vi "MultiChannelFeedbackCooling_aod_feedback(Host)_PIDXYZ.vi"(5 "RIO Device":T1="RIO0") -> ()   [LabVIEW 2016]
doc: "This VI will will initialize the FPGA VI and then continually read and convert single point values from 4 channels of an analog input module."
uses:
  <vilib>/userdefined/High Color/nirio_resource_hc.ctl
  <vilib>/rvi/Analysis/host/Butterworth/config/Butterworth Filter Order.ctl
  <vilib>/rvi/Analysis/host/Butterworth/config/Butterworth Filter Type.ctl
  <vilib>/FPGAPlugInAG/PXIe-7847R/niLvFpga_Open_PXIe-7847R.vi
  <vilib>/FPGAPlugInAG/PXIe-7847R/niLvFpga_Run_PXIe-7847R.vi
  <vilib>/rvi/Analysis/host/Butterworth/config/BwScaledCoefficients.vi
  <vilib>/Utility/error.llb/Error Cluster From Error Code.vi
  <vilib>/rvi/errors/niLvFpgaAdjustHostInterfaceError.vi
  <vilib>/Utility/file.llb/Read From Spreadsheet File (I64).vi
  <vilib>/FPGAPlugInAG/PXIe-7847R/niLvFpga_Close_PXIe-7847R.vi
  <vilib>/rvi/interface/nirviOpenFPGA/nirviOpenFPGA.xnode
  FPGA Bitfiles/Microspherefeedb_FPGATarget_MultiChannelfFee_cW1Hvxk6p+4.lvbitx
  <vilib>/rvi/interface/nirviMethod/nirviMethod.xnode
  <vilib>/rvi/Analysis/host/Butterworth/XNode/ButterworthCoefficients.xnode
  <vilib>/rvi/interface/nirviReadWriteControl/nirviReadWriteControl.xnode
  <vilib>/rvi/interface/nirviCloseFPGA/nirviCloseFPGA.xnode
  NiFpgaLv.dll
  <vilib>/rvi/Analysis/host/Public/NI_FpgaMspHost.lvlib
panel:
  in  "hp freq band imgZ":dbl=5000.0
  in  "lp freq band imgZ":dbl=5000.0
  in  "dg band imgZ":fxp<+/-,24,12>
  in  "hp freq band d2Z":dbl=5000.0
  in  "lp freq band d2Z":dbl=5000.0
  in  "dg band d2Z":fxp<+/-,24,12>
  in  "hp freq bandZ":dbl=49.0
  in  "lp freq bandZ":dbl=45.0
  in  "dg band Z":fxp<+/-,24,12>
  in  "dg band Y":fxp<+/-,24,12>
  in  "hp freq bandY":dbl=5000.0
  in  "lp freq bandY":dbl=5000.0
  in  "hp freq bandX":dbl=5000.0
  in  "lp freq bandX":dbl=5000.0
  in  "dg band X":fxp<+/-,24,12>
  in  "pg 1":fxp<+/-,24,12>
  in  "ig 1":fxp<+/-,24,6>
  in  "pg 0":fxp<+/-,24,12>
  in  "ig 0":fxp<+/-,24,6>
  out "tot_fb_img":i16(graph)
  out "fb_img":i16(graph)
  out "AI_img":i16(graph)=465
  in  "pg_img":fxp<+/-,24,12>
  in  "dg_img":fxp<+/-,24,12>
  in  "ig_img":fxp<+/-,24,6>
  in  "setpt_img":i16=3000
  in  "Upper lim_img":fxp<+/-,16,16>=1000.0
  in  "Lower lim_img":fxp<+/-,16,16>=-1000.0
  in  "lp freq_img":dbl=5000.0
  in  "hp freq_img":dbl=5000.0
  in  "output offset_img":i16
  in  "End value arb (ch1)":fxp<+/-,32,16>
  in  "Step arb (ch1)":fxp<+/-,32,16>=0.0500030517578125
  in  "Arb gain (ch2)":fxp<+/-,24,12>
  in  "z arb scale":fxp<+/-,33,17>=1.0
  in  "ramp arb drive":bool
  in  "End value arb (ch0)":fxp<+/-,32,16>
  in  "Step arb (ch0)":fxp<+/-,32,16>
  in  "Delay Time (s) arb":dbl=0.001 caption="Delay Time (s)"
  in  "Buffer file path":path=path "C:/Users/UsphereLab/Documents/GitHub/Optlev/scriptssiny_buffer.txt"
  in  "Write data to buffers":bool
  in  "Arb steps per cycle":u16=50
  in  "Arb gain (ch1)":fxp<+/-,24,12>
  in  "Arb gain (ch0)":fxp<+/-,24,12>
  in  "power setpt":i16
  in  "Upper lim pow":fxp<+/-,16,16>=10000.0
  in  "Lower lim pow":fxp<+/-,16,16>=-10000.0
  in  "hp freq pow":dbl=5000.0
  in  "lp freq pow":dbl=5000.0
  in  "Use_PID2_power":bool
  in  "hp freq 1":dbl=400.0
  in  "hp freq 0":dbl=600.0
  in  "lp freq 0":dbl=600.0
  in  "DC offset 0":i16
  in  "Lower lim 0":fxp<+/-,16,16>=-200.0
  in  "Upper lim 0":fxp<+/-,16,16>=200.0
  in  "Dg 0":fxp<+/-,24,12>
  in  "Bead setpt 0":i16
  in  "change pars":bool
  in  "hp freq 2":dbl=1600.0
  in  "lp freq 1":dbl=400.0
  in  "lp freq 2":dbl=1600.0
  in  "ramp power":bool
  in  "End value power":i16=-500
  in  "Step power":i16=1
  in  "Delay Time (s) power":dbl=0.01 caption="Delay Time (s)"
  in  "Count(usec)":u32=10
  in  "?":u16(ring)=2 items=["Both", "AOD", "Bead"]
  in  "?":u16(ring)=2 items=["Both", "AOD", "Bead"]
  in  "?":u16(ring) items=["Both", "AOD", "Bead"]
  in  "?":u16(ring)=2 items=["Both", "AOD", "Bead"]
  in  "?":u16(ring)=1 items=["Both", "AOD", "Bead"]
  in  "?":u16(ring)=2 items=["Both", "AOD", "Bead"]
  in  "Pg d2":fxp<+/-,24,12>=-6.0
  in  "Ig d2":fxp<+/-,24,6>=-0.7999992370605469
  in  "Dg d2":fxp<+/-,24,12>
  in  "Ig 2":fxp<+/-,24,6>
  in  "DC offset 2":i16=2200
  in  "Lower lim 2":fxp<+/-,16,16>=-20.0
  in  "Upper lim 2":fxp<+/-,16,16>=1500.0
  in  "Dg 2":fxp<+/-,24,12>
  in  "Pg 2":fxp<+/-,24,12>
  in  "Bead setpt 2":i16
  in  "change pars 2":bool
  in  "change pars 1":bool
  in  "DC offset 1":i16
  in  "Lower lim 1":fxp<+/-,16,16>=-200.0
  in  "Upper lim 1":fxp<+/-,16,16>=200.0
  in  "Dg 1":fxp<+/-,24,12>
  in  "Bead setpt 1":i16
  out "Tot feedback + DC, Ch2":i16(graph)=2200
  out "Individual feedback, Ch2":cluster{"fb_0":i16, "fb_d0":i16}(graph)
  out "AI1 2":cluster{"AI2":i16, "AI5":i16}(graph)={"AI2"=-987, "AI5"=-987}
  out "Tot feedback + DC, Ch1":i16(graph)
  out "Individual feedback, Ch1":cluster{"fb_0":i16, "fb_d0":i16}(graph)
  out "AI1":cluster{"AI1":i16, "AI4":i16}(graph)={"AI1"=-51, "AI4"=-51}
  out "Tot feedback + DC, Ch0":i16(graph)
  out "Individual feedback, Ch0":cluster{"fb_0":i16, "fb_d0":i16}(graph)
  out "AI0":cluster{"AI0":i16, "AI3":i16}(graph)={"AI0"=-20, "AI3"=-20}
  in  "stop":bool
  # "FPGA feedback GUI"
  # "Bead arbitrary drive:"
  # "PID controls, X (ch 0):"
  # "Bead feedback:"
  # "PID controls, Y (ch 1):"
  # "Bead feedback:"
  # "PID controls, Z (ch 2):"
  # "Bead feedback:"
  # "AOD feeback:"
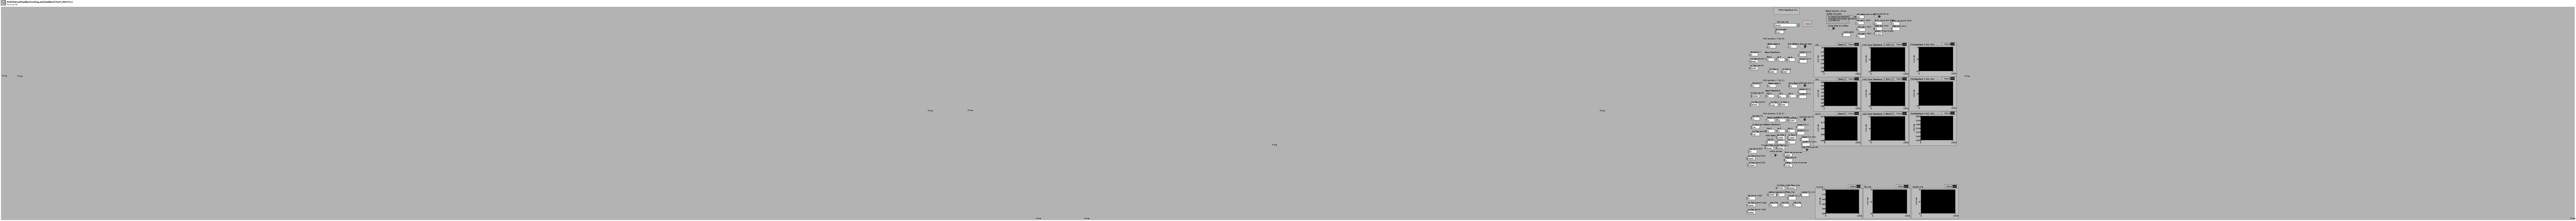
[diagram p1: front panel]
types:
  T1 = typedef "nirio_resource_hc.ctl" = tag
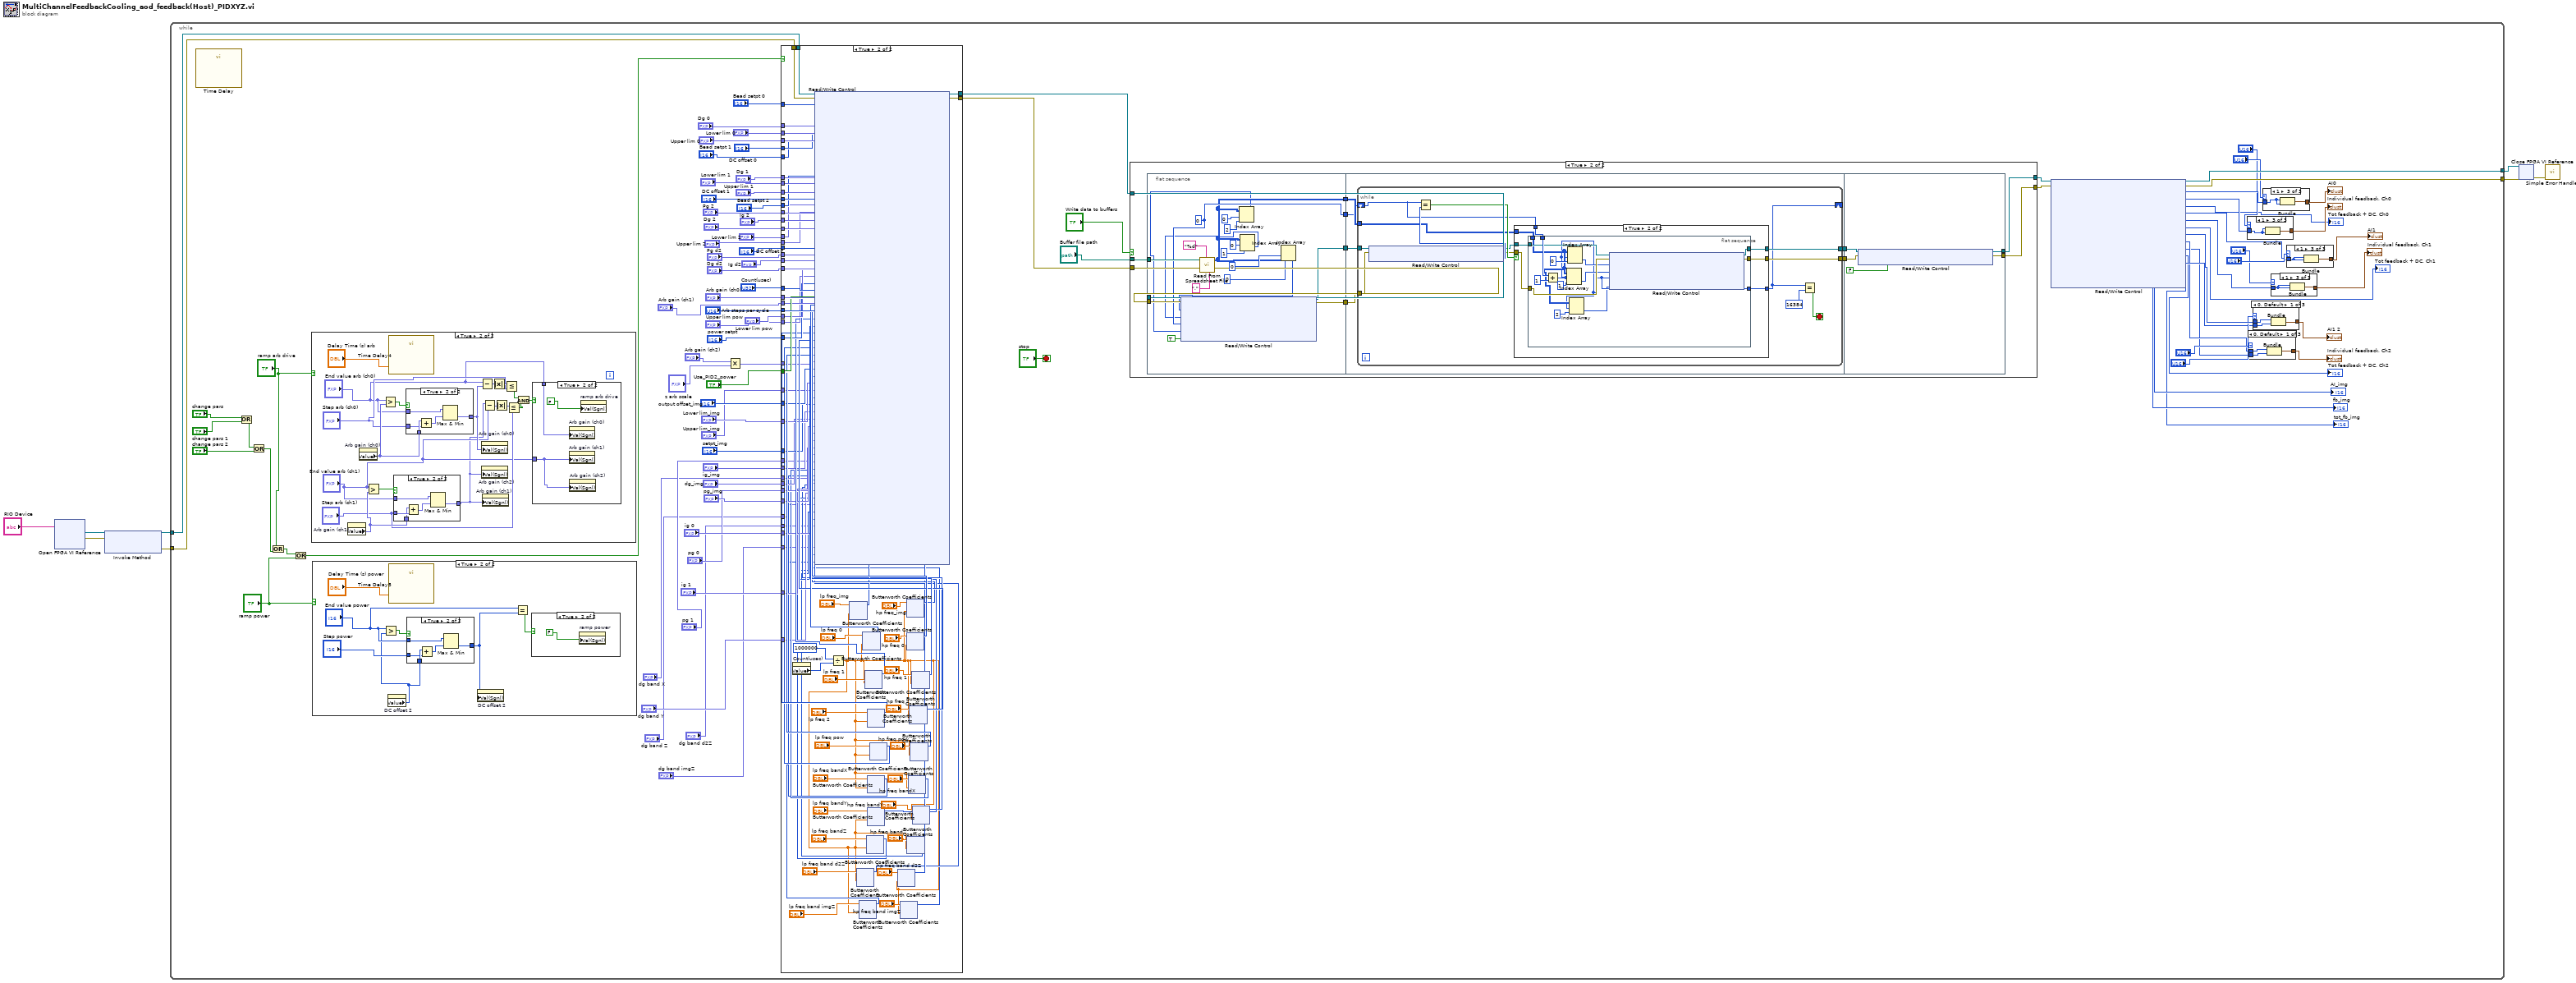
[diagram p0: block diagram]
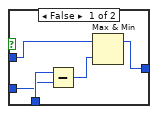
[diagram p4: hidden frame]
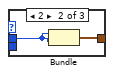
[diagram p5: hidden frame]
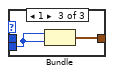
[diagram p6: hidden frame]
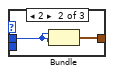
[diagram p7: hidden frame]
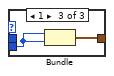
[diagram p8: hidden frame]
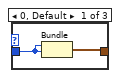
[diagram p9: hidden frame]
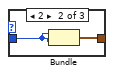
[diagram p10: hidden frame]
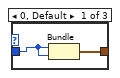
[diagram p11: hidden frame]
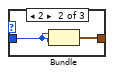
[diagram p12: hidden frame]
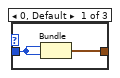
[diagram p13: hidden frame]
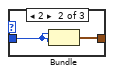
[diagram p14: hidden frame]
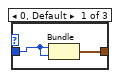
[diagram p15: hidden frame]
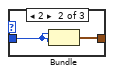
[diagram p16: hidden frame]
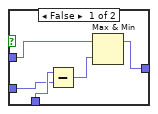
[diagram p18: hidden frame]
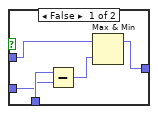
[diagram p20: hidden frame]
diagram:
  n1 = xnode "Open FPGA VI Reference"("resource name"="RIO Device") -> ("FPGA VI Reference Out"=w3:refnum<k20>, "error out"=w2:errorcluster)  [unwired: 1 in]
  n2 = xnode "Invoke Method"("FPGA VI Reference In"=w3, "error in"=w2) -> ("FPGA VI Reference Out"=w5:refnum<k20>, "error out"=w4:errorcluster)  [unwired: 1 in]
  n3 = while {
    tunnel: [w101] -> w8
    tunnel: w5 -> [w93]
    tunnel: w4 -> [w92]
    tunnel: [w100] -> w1
    stop <- "stop" stop-if-true
    n4 = call "Time Delay"() -> ()  [unwired: 11 in, 1 out]
    n5 = Or(x="change pars", y="change pars 1") -> (x .or. y?=w66:bool)
    n6 = Or(x=w66, y="change pars 2") -> (x .or. y?=w32:bool)
    n7 = Or(x="ramp arb drive", y=w32) -> (x .or. y?=w39:bool)
    n8 = Or(x=w39, y="ramp power") -> (x .or. y?=w40:bool)
    n9 = case shown="True" "ramp arb drive" {
      frame False {
      }
      frame True {
        n10 = property on="Arb gain (ch1)" class="DigNum (strict)"() -> ("Value"=w171:fxp<+/-,24,12>)  [unwired: 2 in, 2 out]
        n11 = property on="Arb gain (ch0)" class="DigNum (strict)"() -> ("Value"=w174:fxp<+/-,24,12>)  [unwired: 2 in, 2 out]
        n12 = Greater?(x="End value arb (ch1)", y=w171) -> (0:w172:bool)
        n13 = Greater?(x="End value arb (ch0)", y=w174) -> (0:w175:bool)
        n14 = call "Time Delay4"("Delay Time (s)"="Delay Time (s) arb") -> ()  [unwired: 10 in, 1 out]
        n15 = case shown="True" w172 {
          tunnel: "End value arb (ch1)" -> [w177 w183]
          tunnel: w171 -> [w180 w181]
          tunnel: "Step arb (ch1)" -> [w179 w185]
          tunnel: [w176 w182] -> w158
          frame False {
            n16 = Subtract(x=w180, y=w179) -> (x-y=w178:fxp<+/-,33,17>)
            n17 = Max & Min(x=w177, y=w178) -> (max(x,y)=w176:fxp<+/-,33,17>)  [unwired: 1 out]
          }
          frame True {
            n18 = Add(x=w181, y=w185) -> (x+y=w184:fxp<+/-,33,17>)
            n19 = Max & Min(x=w183, y=w184) -> (min(x,y)=w182:fxp<+/-,33,17>)  [unwired: 1 out]
          }
        }
        n20 = case shown="True" w175 {
          tunnel: "End value arb (ch0)" -> [w190 w195]
          tunnel: w174 -> [w193 w198]
          tunnel: "Step arb (ch0)" -> [w192 w197]
          tunnel: [w189 w194] -> w170
          frame False {
            n21 = Subtract(x=w193, y=w192) -> (x-y=w191:fxp<+/-,33,17>)
            n22 = Max & Min(x=w190, y=w191) -> (max(x,y)=w189:fxp<+/-,33,17>)  [unwired: 1 out]
          }
          frame True {
            n23 = Add(x=w198, y=w197) -> (x+y=w196:fxp<+/-,33,17>)
            n24 = Max & Min(x=w195, y=w196) -> (min(x,y)=w194:fxp<+/-,33,17>)  [unwired: 1 out]
          }
        }
        n25 = Subtract(x="End value arb (ch0)", y=w170) -> (x-y=w169:fxp<+/-,34,18>)
        n26 = property on="Arb gain (ch0)" class="DigNum (strict)"("Val(Sgnl)"=w170) -> ()  [unwired: 2 in, 2 out]
        n27 = property on="Arb gain (ch2)" class="DigNum (strict)"("Val(Sgnl)"=w158) -> ()  [unwired: 2 in, 2 out]
        n28 = Subtract(x=w158, y="End value arb (ch1)") -> (x-y=w166:fxp<+/-,34,18>)
        n29 = property on="Arb gain (ch1)" class="DigNum (strict)"("Val(Sgnl)"=w158) -> ()  [unwired: 2 in, 2 out]
        n30 = Absolute Value(x=w169) -> (abs(x)=w168:fxp<+,33,17>)
        n31 = Absolute Value(x=w166) -> (abs(x)=w165:fxp<+,33,17>)
        n32 = Less Or Equal?(x=w168, y="Step arb (ch0)") -> (x <= y?=w162:bool)
        n33 = Less Or Equal?(x=w165, y="Step arb (ch1)") -> (x <= y?=w161:bool)
        n34 = And(x=w162, y=w161) -> (x .and. y?=w163:bool)
        n35 = case shown="True" w163 {
          tunnel: "End value arb (ch0)" -> [_ w187]
          tunnel: "End value arb (ch1)" -> [_ w186]
          frame False {
          }
          frame True {
            n36 = property on="Arb gain (ch0)" class="DigNum (strict)"("Val(Sgnl)"=w187) -> ()  [unwired: 2 in, 2 out]
            n37 = property on="Arb gain (ch1)" class="DigNum (strict)"("Val(Sgnl)"=w186) -> ()  [unwired: 2 in, 2 out]
            n38 = property on="Arb gain (ch2)" class="DigNum (strict)"("Val(Sgnl)"=w186) -> ()  [unwired: 2 in, 2 out]
            n39 = property on="ramp arb drive" class="Bool (strict)"("Val(Sgnl)"=FALSE) -> ()  [unwired: 2 in, 2 out]
          }
        }
      }
    }
    n40 = case shown="True" "ramp power" {
      frame False {
      }
      frame True {
        n41 = property on="DC offset 2" class="DigNum (strict)"() -> ("Value"=w103:i16)  [unwired: 2 in, 2 out]
        n42 = Greater?(x="End value power", y=w103) -> (0:w108:bool)
        n43 = call "Time Delay5"("Delay Time (s)"="Delay Time (s) power") -> ()  [unwired: 10 in, 1 out]
        n44 = case shown="True" w108 {
          tunnel: "End value power" -> [w111 w116]
          tunnel: w103 -> [w114 w119]
          tunnel: "Step power" -> [w113 w118]
          tunnel: [w110 w115] -> w102
          frame False {
            n45 = Subtract(x=w114, y=w113) -> (x-y=w112:i16)
            n46 = Max & Min(x=w111, y=w112) -> (max(x,y)=w110:i16)  [unwired: 1 out]
          }
          frame True {
            n47 = Add(x=w119, y=w118) -> (x+y=w117:i16)
            n48 = Max & Min(x=w116, y=w117) -> (min(x,y)=w115:i16)  [unwired: 1 out]
          }
        }
        n49 = property on="DC offset 2" class="DigNum (strict)"("Val(Sgnl)"=w102) -> ()  [unwired: 2 in, 2 out]
        n50 = Equal?(x="End value power", y=w102) -> (x = y?=w107:bool)
        n51 = case shown="True" w107 {
          frame False {
          }
          frame True {
            n52 = property on="ramp power" class="Bool (strict)"("Val(Sgnl)"=FALSE) -> ()  [unwired: 2 in, 2 out]
          }
        }
      }
    }
    n53 = Multiply(x="Arb gain (ch2)", y="z arb scale") -> (x*y=w29:fxp<+/-,56,28>)
    n54 = case shown="True" w40 {
      tunnel: w92 -> [w280 w364]
      tunnel: [w280 w372] -> w88
      tunnel: [w279 w371] -> w89
      tunnel: "Bead setpt 0" -> [_ w370]
      tunnel: "Dg 0" -> [_ w369]
      tunnel: "Upper lim 0" -> [_ w367]
      tunnel: "Lower lim 0" -> [_ w368]
      tunnel: "DC offset 0" -> [_ w366]
      tunnel: w93 -> [w279 w365]
      tunnel: "Bead setpt 1" -> [_ w363]
      tunnel: "Dg 1" -> [_ w362]
      tunnel: "Lower lim 1" -> [_ w361]
      tunnel: "Upper lim 1" -> [_ w360]
      tunnel: "DC offset 1" -> [_ w359]
      tunnel: "Bead setpt 2" -> [_ w358]
      tunnel: "Pg 2" -> [_ w357]
      tunnel: "Ig 2" -> [_ w356]
      tunnel: "Dg 2" -> [_ w355]
      tunnel: "Lower lim 2" -> [_ w354]
      tunnel: "Upper lim 2" -> [_ w353]
      tunnel: "DC offset 2" -> [_ w352]
      tunnel: "Pg d2" -> [_ w351]
      tunnel: "Ig d2" -> [_ w350]
      tunnel: "Dg d2" -> [_ w349]
      tunnel: "Arb gain (ch0)" -> [_ w348]
      tunnel: "Arb gain (ch1)" -> [_ w334]
      tunnel: "Arb steps per cycle" -> [_ w347]
      tunnel: "Count(usec)" -> [_ w346]
      tunnel: "Use_PID2_power" -> [_ w337]
      tunnel: "Lower lim pow" -> [_ w333]
      tunnel: "Upper lim pow" -> [_ w332]
      tunnel: "power setpt" -> [_ w331]
      tunnel: w29 -> [_ w322]
      tunnel: "output offset_img" -> [_ w321]
      tunnel: "Lower lim_img" -> [_ w317]
      tunnel: "Upper lim_img" -> [_ w316]
      tunnel: "setpt_img" -> [_ w314]
      tunnel: "ig_img" -> [_ w313]
      tunnel: "dg_img" -> [_ w312]
      tunnel: "pg_img" -> [_ w311]
      tunnel: "ig 0" -> [_ w310]
      tunnel: "pg 0" -> [_ w309]
      tunnel: "ig 1" -> [_ w308]
      tunnel: "pg 1" -> [_ w307]
      tunnel: "dg band X" -> [_ w306]
      tunnel: "dg band Y" -> [_ w299]
      tunnel: "dg band Z" -> [_ w296]
      tunnel: "dg band d2Z" -> [_ w291]
      tunnel: "dg band imgZ" -> [_ w286]
      frame False {
      }
      frame True {
        n55 = property on="Count(usec)" class="DigNum (strict)"() -> ("Value"=w342:u32)  [unwired: 2 in, 2 out]
        n56 = Divide(x=u32 1000000, y=w342) -> (x/y=w281:dbl)
        n57 = xnode "Butterworth Coefficients"("cutoff frequency (Hz)"="lp freq_img", "sample rate (S/s)"=w281) -> ("scaled coefficients"=w315:i32[])  [unwired: 1 in, 1 out]
        n58 = xnode "Butterworth Coefficients"("cutoff frequency (Hz)"="lp freq band d2Z", "sample rate (S/s)"=w281) -> ("scaled coefficients"=w287:i32[])  [unwired: 1 in, 1 out]
        n59 = xnode "Butterworth Coefficients"("cutoff frequency (Hz)"="lp freq band imgZ", "sample rate (S/s)"=w281) -> ("scaled coefficients"=w284:i32[])  [unwired: 1 in, 1 out]
        n60 = xnode "Butterworth Coefficients"("cutoff frequency (Hz)"="lp freq 0", "sample rate (S/s)"=w281) -> ("scaled coefficients"=w330:i32[])  [unwired: 1 in, 1 out]
        n61 = xnode "Butterworth Coefficients"("cutoff frequency (Hz)"="lp freq 1", "sample rate (S/s)"=w281) -> ("scaled coefficients"=w328:i32[])  [unwired: 1 in, 1 out]
        n62 = xnode "Butterworth Coefficients"("cutoff frequency (Hz)"="lp freq bandZ", "sample rate (S/s)"=w281) -> ("scaled coefficients"=w292:i32[])  [unwired: 1 in, 1 out]
        n63 = xnode "Butterworth Coefficients"("cutoff frequency (Hz)"="lp freq 2", "sample rate (S/s)"=w281) -> ("scaled coefficients"=w326:i32[])  [unwired: 1 in, 1 out]
        n64 = xnode "Butterworth Coefficients"("cutoff frequency (Hz)"="lp freq bandX", "sample rate (S/s)"=w281) -> ("scaled coefficients"=w302:i32[])  [unwired: 1 in, 1 out]
        n65 = xnode "Butterworth Coefficients"("cutoff frequency (Hz)"="lp freq bandY", "sample rate (S/s)"=w281) -> ("scaled coefficients"=w298:i32[])  [unwired: 1 in, 1 out]
        n66 = xnode "Butterworth Coefficients"("cutoff frequency (Hz)"="lp freq pow", "sample rate (S/s)"=w281) -> ("scaled coefficients"=w324:i32[])  [unwired: 1 in, 1 out]
        n67 = xnode "Butterworth Coefficients"("cutoff frequency (Hz)"="hp freq band d2Z", "sample rate (S/s)"=w281) -> ("scaled coefficients"=w288:i32[])  [unwired: 1 in, 1 out]
        n68 = xnode "Butterworth Coefficients"("cutoff frequency (Hz)"="hp freq band imgZ", "sample rate (S/s)"=w281) -> ("scaled coefficients"=w285:i32[])  [unwired: 1 in, 1 out]
        n69 = xnode "Butterworth Coefficients"("cutoff frequency (Hz)"="hp freq_img", "sample rate (S/s)"=w281) -> ("scaled coefficients"=w318:i32[])  [unwired: 1 in, 1 out]
        n70 = xnode "Butterworth Coefficients"("cutoff frequency (Hz)"="hp freq 0", "sample rate (S/s)"=w281) -> ("scaled coefficients"=w329:i32[])  [unwired: 1 in, 1 out]
        n71 = xnode "Butterworth Coefficients"("cutoff frequency (Hz)"="hp freq bandZ", "sample rate (S/s)"=w281) -> ("scaled coefficients"=w293:i32[])  [unwired: 1 in, 1 out]
        n72 = xnode "Butterworth Coefficients"("cutoff frequency (Hz)"="hp freq bandX", "sample rate (S/s)"=w281) -> ("scaled coefficients"=w303:i32[])  [unwired: 1 in, 1 out]
        n73 = xnode "Butterworth Coefficients"("cutoff frequency (Hz)"="hp freq 2", "sample rate (S/s)"=w281) -> ("scaled coefficients"=w325:i32[])  [unwired: 1 in, 1 out]
        n74 = xnode "Butterworth Coefficients"("cutoff frequency (Hz)"="hp freq pow", "sample rate (S/s)"=w281) -> ("scaled coefficients"=w323:i32[])  [unwired: 1 in, 1 out]
        n75 = xnode "Butterworth Coefficients"("cutoff frequency (Hz)"="hp freq 1", "sample rate (S/s)"=w281) -> ("scaled coefficients"=w327:i32[])  [unwired: 1 in, 1 out]
        n76 = xnode "Butterworth Coefficients"("cutoff frequency (Hz)"="hp freq bandY", "sample rate (S/s)"=w281) -> ("scaled coefficients"=w297:i32[])  [unwired: 1 in, 1 out]
        n77 = xnode "Read/Write Control"("FPGA VI Reference In"=w365, "error in"=w364, "Dc Pos 0"=w370, "dg 0"=w369, "Lower lim 0"=w368, "Upper lim 0"=w367, "output offset 0"=w366, "Dc Pos 1"=w363, "dg 1"=w362, "Lower lim 1"=w361, "Upper lim 1"=w360, "output offset 1"=w359, "Dc Pos 2"=w358, "pg 2"=w357, "ig 3"=w356, "dg 2"=w355, "Lower lim 2"=w354, "Upper lim 2"=w353, "output offset 2"=w352, "pg d0 3"=w351, "ig d03"=w350, "dg d0 3"=w349, "Arb gain (ch0)"=w348, "Arb gain (ch1)"=w334, "Arb steps per cycle"=w347, "Lower lim 4"=w333, "Upper lim d0 3"=w332, "Dc Pos d2"=w331, "Count(uSec)"=w346, "Use_PID2_X 2"=w337, "lp coeff 0"=w330, "hp coeff 0"=w329, "lp coeff 1"=w328, "hp coeff 1"=w327, "lp coeff 2"=w326, "hp coeff 2"=w325, "lp coeff d2"=w324, "hp coeff d2"=w323, "Arb gain (ch2)"=w322, "output offset_img"=w321, "hp coeff_img"=w318, "Lower lim_img"=w317, "Upper lim_img"=w316, "lp coeff_img"=w315, "setpt_img"=w314, "ig_img"=w313, "dg_img"=w312, "pg_img"=w311, "ig 0"=w310, "pg 0"=w309, "ig 1"=w308, "pg 1"=w307, "dg band X"=w306, "hp coeff band X"=w303, "lp coeff band X"=w302, "dg band Y"=w299, "hp coeff band Y"=w297, "lp coeff band Y"=w298, "dg band Z"=w296, "hp coeff band Z"=w293, "lp coeff band Z"=w292, "dg band dZ"=w291, "hp coeff band dZ"=w288, "lp coeff band dZ"=w287, "dg band imgZ"=w286, "hp coeff band imgZ"=w285, "lp coeff band imgZ"=w284) -> ("FPGA VI Reference Out"=w371:refnum<k20>, "error out"=w372:errorcluster)
      }
    }
    n78 = case shown="True" "Write data to buffers" {
      tunnel: "Buffer file path" -> [_ w211]
      tunnel: w89 -> [w200 w210]
      tunnel: w88 -> [w199 w209]
      tunnel: [w200 w202] -> w87
      tunnel: [w199 w201] -> w86
      frame False {
      }
      frame True {
        n79 = flat-sequence {
          tunnel: w211 -> [w230]
          tunnel: w210 -> [w228]
          tunnel: w209 -> [w227]
          tunnel: [w222] -> w208
          tunnel: [w221] -> w207
          tunnel: [w215] -> w206
          tunnel: [w220] -> w205
          tunnel: w208 -> [w236]
          tunnel: w207 -> [w235]
          tunnel: w206 -> [w234]
          tunnel: w205 -> [w233]
          tunnel: [w232] -> w204
          tunnel: [w231] -> w203
          tunnel: w204 -> [w278]
          tunnel: w203 -> [w277]
          tunnel: [w276] -> w202
          tunnel: [w275] -> w201
          frame #0 {
            w220 = 0
            n80 = call-poly <vilib>:"Read From Spreadsheet File.vi"("delimiter (\\t)"="," ("delimiter (\\t)"), "format (%d)"="%d", "file path (dialog if empty)"=w230) -> ("all rows"=w215:i64[][])  [unwired: 4 in, 4 out]
            n81 = Index Array(array=w215, index (row)=0, index (col)=2 ("disabled index (col)")) -> (element=w212:i64)
            n82 = Index Array(array=w215, index (row)=0, index (col)=1 ("disabled index (col)")) -> (element=w218:i64)
            n83 = Index Array(array=w215, index (row)=0, index (col)=0 ("disabled index (col)")) -> (element=w219:i64)
            n84 = xnode "Read/Write Control"("FPGA VI Reference In"=w228, "error in"=w227, "data_buffer_1"=w219, "data_buffer2"=w218, "write_address"=w220, "data_buffer3"=w212, "ready_to_write"=TRUE) -> ("FPGA VI Reference Out"=w221:refnum<k20>, "error out"=w222:errorcluster)
          }
          frame #1 {
            n85 = while {
              shift-right: [w237] -> _
              shift-left: w233 -> [w245]
              tunnel: w235 -> [w249]
              tunnel: w236 -> [w248]
              tunnel: w234 -> [w244]
              tunnel: [w239] -> w232
              tunnel: [w238] -> w231
              stop <- w240 stop-if-true
              n86 = xnode "Read/Write Control"("FPGA VI Reference In"=w249, "error in"=w248) -> ("FPGA VI Reference Out"=w243:refnum<k20>, "error out"=w242:errorcluster, "written_address"=w247:u32)
              n87 = Equal?(x=w245, y=w247) -> (x = y?=w246:bool)
              n88 = case shown="True" w246 {
                tunnel: w245 -> [w252 w259]
                tunnel: w244 -> [_ w258]
                tunnel: w243 -> [w251 w257]
                tunnel: w242 -> [w250 w256]
                tunnel: [w252 w255] -> w237
                tunnel: [w251 w254] -> w239
                tunnel: [w250 w253] -> w238
                frame False {
                }
                frame True {
                  n89 = flat-sequence {
                    tunnel: w259 -> [w272]
                    tunnel: w258 -> [w262]
                    tunnel: w257 -> [w269]
                    tunnel: w256 -> [w268]
                    tunnel: [w261] -> w255
                    tunnel: [w266] -> w254
                    tunnel: [w265] -> w253
                    frame #0 {
                      n90 = Add(x=w272, y=1) -> (x+y=w261:i32)
                      n91 = Index Array(array=w262, index (row)=w261, index (col)=1 ("disabled index (col)")) -> (element=w267:i64)
                      n92 = Index Array(array=w262, index (row)=w261, index (col)=0 ("disabled index (col)")) -> (element=w264:i64)
                      n93 = Index Array(array=w262, index (row)=w261, index (col)=2) -> (element=w260:i64)
                      n94 = xnode "Read/Write Control"("FPGA VI Reference In"=w269, "error in"=w268, "data_buffer_1"=w264, "data_buffer2"=w267, "write_address"=w261, "data_buffer3"=w260) -> ("FPGA VI Reference Out"=w266:refnum<k20>, "error out"=w265:errorcluster)
                    }
                  }
                }
              }
              n95 = Equal?(x=w237, y=u16 16384) -> (x = y?=w240:bool)
            }
          }
          frame #2 {
            n96 = xnode "Read/Write Control"("FPGA VI Reference In"=w278, "error in"=w277, "ready_to_write"=FALSE) -> ("FPGA VI Reference Out"=w276:refnum<k20>, "error out"=w275:errorcluster)
          }
        }
      }
    }
    n97 = xnode "Read/Write Control"("FPGA VI Reference In"=w87, "error in"=w86) -> ("FPGA VI Reference Out"=w101:refnum<k20>, "error out"=w100:errorcluster, "AI0"=w63:i16, "fb_0"=w58:i16, "tot_fb_0"=→"Tot feedback + DC, Ch0":i16, "AI1"=w55:i16, "fb_1"=w53:i16, "tot_fb_1"=→"Tot feedback + DC, Ch1":i16, "AI2"=w50:i16, "fb_2"=w46:i16, "fb_d2"=w45:i16, "tot_fb_2"=→"Tot feedback + DC, Ch2":i16, "AI5"=w47:i16, "AI_img"=→"AI_img":i16, "fb_img"=→"fb_img":i16, "tot_fb_img"=→"tot_fb_img":i16)
    n98 = case shown="1" "?" {
      tunnel: w58 -> [w147 w148 w151]
      tunnel: [w146 w149 w150] -> w60
      frame 0, Default {
        n99 = Bundle("fb_0"=w147, "fb_0"=w147) -> (w146:cluster{"fb_0":i16, "fb_0":i16})  [unwired: 1 in]
      }
      frame 2 {
        n100 = Bundle("fb_0"=w148, "fb_0"=w148) -> (w149:cluster{"fb_0":i16, "fb_0":i16})  [unwired: 1 in]
      }
      frame 1 {
        n101 = Bundle("fb_0"=w151, "fb_0"=w151) -> (w150:cluster{"fb_0":i16, "fb_0":i16})  [unwired: 1 in]
      }
    }
    "Individual feedback, Ch0" <- w60
    n102 = case shown="0, Default" "?" {
      tunnel: w46 -> [w122 w123 _]
      tunnel: w45 -> [w121 _ w126]
      tunnel: [w120 w124 w125] -> w43
      frame 0, Default {
        n103 = Bundle("fb_2"=w122, "fb_d2"=w121) -> (w120:cluster{"fb_2":i16, "fb_d2":i16})  [unwired: 1 in]
      }
      frame 2 {
        n104 = Bundle("fb_2"=w123, "fb_2"=w123) -> (w124:cluster{"fb_2":i16, "fb_2":i16})  [unwired: 1 in]
      }
      frame 1 {
        n105 = Bundle("fb_d2"=w126, "fb_d2"=w126) -> (w125:cluster{"fb_d2":i16, "fb_d2":i16})  [unwired: 1 in]
      }
    }
    "Individual feedback, Ch2" <- w43
    n106 = case shown="0, Default" "?" {
      tunnel: w50 -> [w129 w130 _]
      tunnel: w47 -> [w128 _ w133]
      tunnel: [w127 w131 w132] -> w42
      frame 0, Default {
        n107 = Bundle("AI2"=w129, "AI5"=w128) -> (w127:cluster{"AI2":i16, "AI5":i16})  [unwired: 1 in]
      }
      frame 2 {
        n108 = Bundle("AI2"=w130, "AI2"=w130) -> (w131:cluster{"AI2":i16, "AI2":i16})  [unwired: 1 in]
      }
      frame 1 {
        n109 = Bundle("AI5"=w133, "AI5"=w133) -> (w132:cluster{"AI5":i16, "AI5":i16})  [unwired: 1 in]
      }
    }
    "AI1 2" <- w42
    n110 = case shown="1" "?" {
      tunnel: w63 -> [w153 w154 w157]
      tunnel: [w152 w155 w156] -> w62
      frame 0, Default {
        n111 = Bundle("AI0"=w153, "AI0"=w153) -> (w152:cluster{"AI0":i16, "AI0":i16})  [unwired: 1 in]
      }
      frame 2 {
        n112 = Bundle("AI0"=w154, "AI0"=w154) -> (w155:cluster{"AI0":i16, "AI0":i16})  [unwired: 1 in]
      }
      frame 1 {
        n113 = Bundle("AI0"=w157, "AI0"=w157) -> (w156:cluster{"AI0":i16, "AI0":i16})  [unwired: 1 in]
      }
    }
    "AI0" <- w62
    n114 = case shown="1" "?" {
      tunnel: w53 -> [w134 w136 w139]
      tunnel: [w135 w137 w138] -> w52
      frame 0, Default {
        n115 = Bundle("fb_1"=w134, "fb_1"=w134) -> (w135:cluster{"fb_1":i16, "fb_1":i16})  [unwired: 1 in]
      }
      frame 2 {
        n116 = Bundle("fb_1"=w136, "fb_1"=w136) -> (w137:cluster{"fb_1":i16, "fb_1":i16})  [unwired: 1 in]
      }
      frame 1 {
        n117 = Bundle("fb_1"=w139, "fb_1"=w139) -> (w138:cluster{"fb_1":i16, "fb_1":i16})  [unwired: 1 in]
      }
    }
    "Individual feedback, Ch1" <- w52
    n118 = case shown="1" "?" {
      tunnel: w55 -> [w140 w142 w144]
      tunnel: [w141 w143 w145] -> w41
      frame 0, Default {
        n119 = Bundle("AI1"=w140, "AI1"=w140) -> (w141:cluster{"AI1":i16, "AI1":i16})  [unwired: 1 in]
      }
      frame 2 {
        n120 = Bundle("AI1"=w142, "AI1"=w142) -> (w143:cluster{"AI1":i16, "AI1":i16})  [unwired: 1 in]
      }
      frame 1 {
        n121 = Bundle("AI1"=w144, "AI1"=w144) -> (w145:cluster{"AI1":i16, "AI1":i16})  [unwired: 1 in]
      }
    }
    "AI1" <- w41
  }
  n122 = xnode "Close FPGA VI Reference"("FPGA VI Reference In"=w8, "error in"=w1) -> ("error out"=w7:errorcluster)
  n123 = call <vilib>:"Simple Error Handler.vi"("error in (no error)"=w7) -> ()  [unwired: 4 in, 5 out]
